vi "Latihan 13 (SubVI_1).vi"(0 "F":dbl, 1 "Convert":bool) -> (2 "Celcius":dbl, 3 "Kelvin":dbl, 4 "Reamur":dbl)   [LabVIEW 2021]
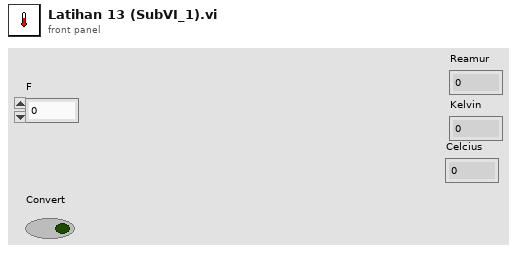
[diagram p1: front panel]
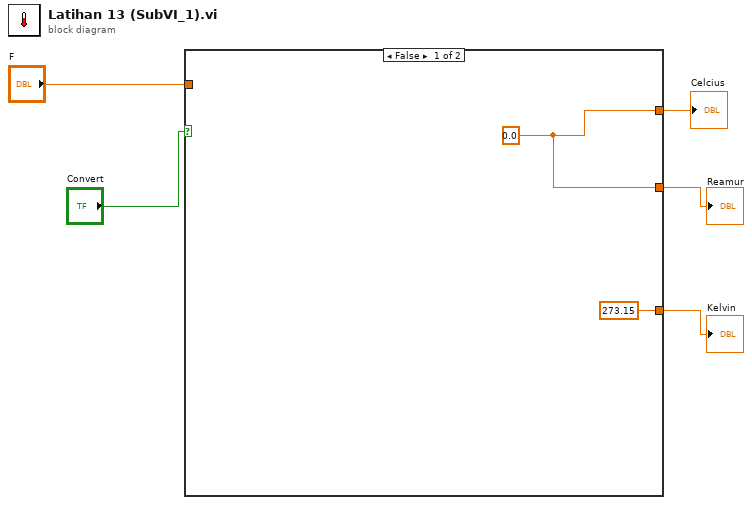
[diagram p0: block diagram]
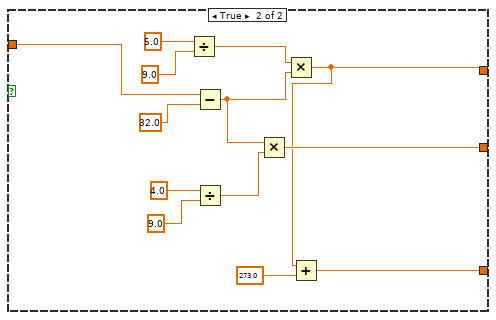
[diagram p2: hidden frame]
diagram:
  n1 = case shown="False" "Convert" {
    tunnel: [w6 w10] -> w4
    tunnel: "F" -> [_ w17]
    tunnel: [w6 w11] -> w2
    tunnel: [273.15 w8] -> w1
    frame False {
      w6 = 0.0
    }
    frame True {
      n2 = Divide(x=5.0, y=9.0) -> (x/y=w16:dbl)
      n3 = Subtract(x=w17, y=32.0) -> (x-y=w13:dbl)
      n4 = Divide(x=4.0, y=9.0) -> (x/y=w12:dbl)
      n5 = Multiply(x=w13, y=w12) -> (x*y=w11:dbl)
      n6 = Multiply(x=w16, y=w13) -> (x*y=w10:dbl)
      n7 = Add(x=w10, y=273.0) -> (x+y=w8:dbl)
    }
  }
  "Celcius" <- w4
  "Reamur" <- w2
  "Kelvin" <- w1
